vi "Check-Temperature-field-settings.vi"(8 "error in":errorcluster, 9 "Correct. params. ref.":refnum<data-value>, 10 "Config. params. ref.":refnum<data-value>, 11 "Temp. params. ref.":refnum<data-value>) -> (0 "error IO":errorcluster, 3 "Passed?":bool)   [LabVIEW 2013, in "CameraVision.lvlib" / "CV-Temperature.lvclass"]
uses:
  CV-Temperature.lvclass
  Configuration/CV-Configuration.lvclass
  Correction/CV-Correction.lvclass
  Correction/CV-Correction.lvclass/CV-Correction.ctl
  Configuration/CV-Configuration.lvclass/CV-Configuration.ctl
  CV-Temperature.lvclass/CV-Temperature.ctl
  Read Temperature field.vi
  Configuration/Read Number of cameras.vi
  Correction/Read 2nd image correlation.vi
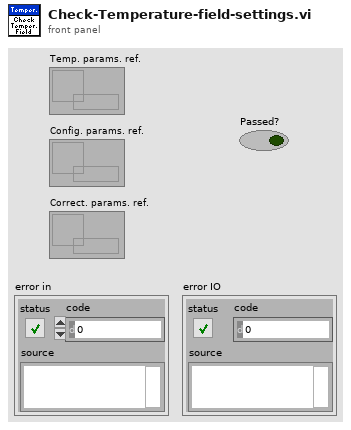
[diagram p1: front panel]
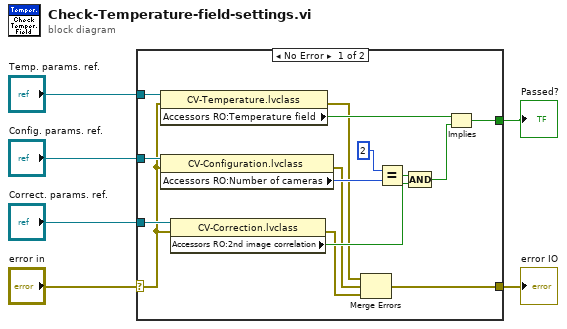
[diagram p0: block diagram]
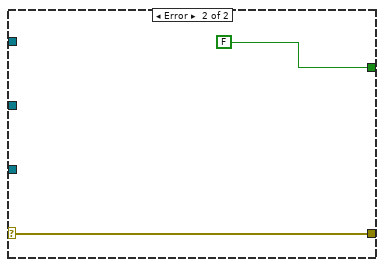
[diagram p2: hidden frame]
diagram:
  n1 = case shown="No Error" "error in" {
    selector: "error in" -> [w7 w22]
    tunnel: "Correct. params. ref." -> [w13 _]
    tunnel: [w8 w22] -> w5
    tunnel: [w20 FALSE] -> w6
    tunnel: "Temp. params. ref." -> [w17 _]
    tunnel: "Config. params. ref." -> [w15 _]
    frame No Error {
      n2 = property class="CV-Temperature.lvclass"(reference=w17, error in=w7) -> (error out=w11:errorcluster, "Accessors RO:Temperature field"=w16:bool)  [unwired: 1 out]
      n3 = property class="CV-Configuration.lvclass"(reference=w15, error in=w7) -> (error out=w10:errorcluster, "Accessors RO:Number of cameras"=w14:i32)  [unwired: 1 out]
      n4 = property class="CV-Correction.lvclass"(reference=w13, error in=w7) -> (error out=w9:errorcluster, "Accessors RO:2nd image correlation"=w12:bool)  [unwired: 1 out]
      n5 = Merge Errors(w11, w10, w9) -> (w8:errorcluster)
      n6 = Equal?(x=2 ("y"), y=w14) -> (x = y?=w18:bool)
      n7 = Compound Arithmetic op=AND(w18, w12) -> (w21:bool)
      n8 = Implies(1:w21, 2:w16) -> (0:w20:bool)
    }
    frame Error {
    }
  }
  "Passed?" <- w6
  "error IO" <- w5
